vi "Process Job.vi"(8 "error in (no error)":errorcluster, 10 "Job":refnum<class>, 11 "Worker In":refnum<class "Worker.lvclass">) -> (0 "error out":errorcluster, 3 "Worker Out":refnum<class "Worker.lvclass">)   [LabVIEW 2020, in "Worker.lvclass"]
uses:
  Worker.lvclass
  <vilib>/Astemes/Triarc Framework/Process/Process.lvclass/Process.ctl
  <vilib>/Astemes/Triarc Framework/Process/Public/Lifecycle/Get Lifecycle State.vi
  <vilib>/Astemes/Triarc Framework/Process/Private/SubVIs/Handle Debug Data.vi
  <vilib>/Utility/error.llb/Clear Errors.vi
  <vilib>/Utility/High Resolution Relative Seconds.vi
  <vilib>/Utility/error.llb/Error Cluster From Error Code.vi
  Worker.lvclass/Worker.ctl
  <vilib>/Astemes/Triarc Framework/Process/Process.lvclass
  C:/Git/astemes-triarc-examples/Coffee Shop/Processes/People/Person/Person.lvclass
  C:/Program Files (x86)/National Instruments/LabVIEW 2020/vi.lib/Astemes/Triarc Framework/View/View.lvclass
  C:/Program Files (x86)/National Instruments/LabVIEW 2020/vi.lib/Astemes/Triarc Framework/Process/Process.lvclass
  C:/Program Files (x86)/National Instruments/LabVIEW 2020/vi.lib/Astemes/Triarc Framework/Base/Base.lvclass
  C:/Program Files (x86)/National Instruments/LabVIEW 2020/vi.lib/Astemes/Triarc Framework/Error Handler Interface/Error Handler Interface.lvclass
  C:/Program Files (x86)/National Instruments/LabVIEW 2020/vi.lib/Astemes/Triarc Framework/Logging/Logging.lvclass
  C:/Git/astemes-triarc-examples/Coffee Shop/Processes/People/Workers/Worker/Worker.lvclass
  C:/Git/astemes-triarc-examples/Coffee Shop/Processes/People/Process Job/Job Handler.lvclass
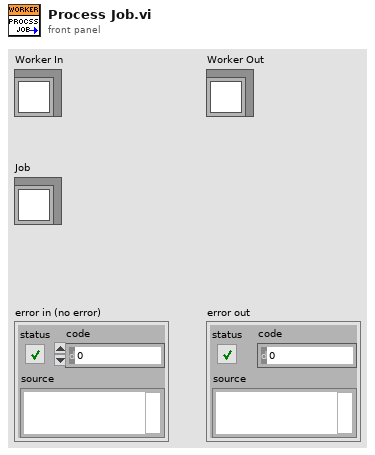
[diagram p1: front panel]
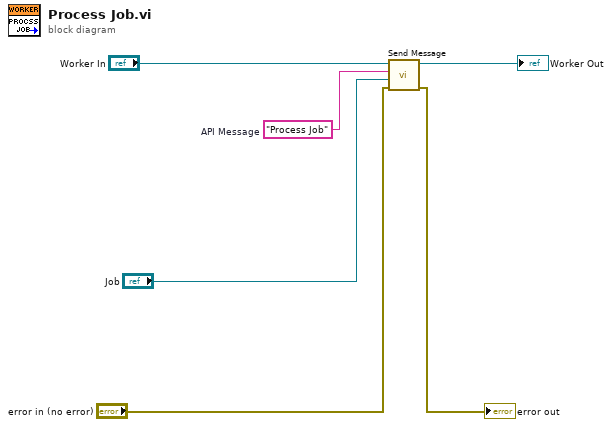
[diagram p0: block diagram]
diagram:
  w3 = "Process Job"  # API Message
  n1 = call <vilib>:"Send Message.vi"("error in (no error)"="error in (no error)", "Message Data"="Job", "Message"=w3, "Process In"="Worker In") -> ("error out"=→"error out":errorcluster, "Process Out"=→"Worker Out":refnum<class "Worker.lvclass">)  [unwired: 6 in]
